vi "Camera.vi"() -> ()   [LabVIEW 2016]
uses:
  <vilib>/rvi/Emulation/niFpgaGetClockAttributes.vi
  <vilib>/rvi/Emulation/niFpgaSctlEmulationGetInTimedLoop.vi
  <vilib>/rvi/Emulation/niFpgaEmulationReportErrorSimple.vi
  <vilib>/rvi/eio/common/nirviEmuTemplateMethod_errors.vi
  <vilib>/rvi/Emulation/niFpgaCriticalErrorInLSC.vi
  <vilib>/eio/EIONode/EIONode.xnode
panel:
  in  "Tlow = t":i16=9
  in  "Fly View Frame Rate = R":i16=10
  in  "Arena View Frame Rate = R":i16=200
  out "Camera flash time":i16
  in  "Camera flash time t":i16
  in  "Flash":bool
  # "** Frequency  = 1 / (Fly View R * 0.0001)   i.e R = 10, Frequency = 1000Hz"
  # "**T period = R*100µs,      T low = t*100 µs"
  # "** Frequency  = 1 / (R * 0.0001)   i.e R = 100, Frequency = 100Hz"
  # "** Trigger the fluorenscence camera (Arena View R - x ) *100 microseconds earlier\n      i.e Arena View R = 100, x = 98,\n           offset x = (100 - 98) * 100 µs = 200 µs"
  # "** Camera flash time is set to be the time for triggering the flash at the end of every video.\n** The unit is second."
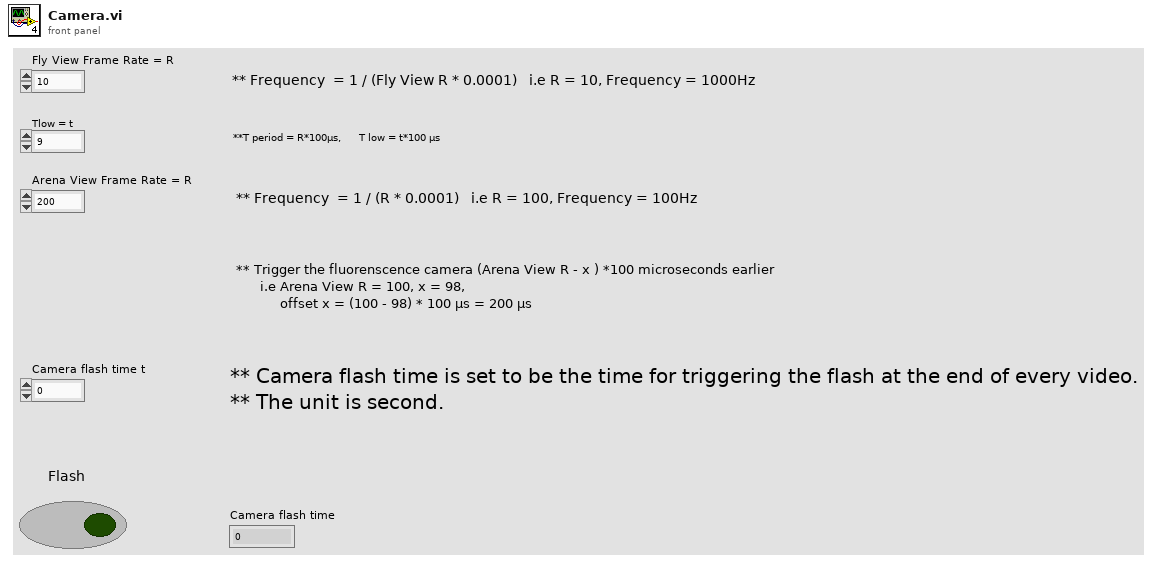
[diagram p1: front panel]
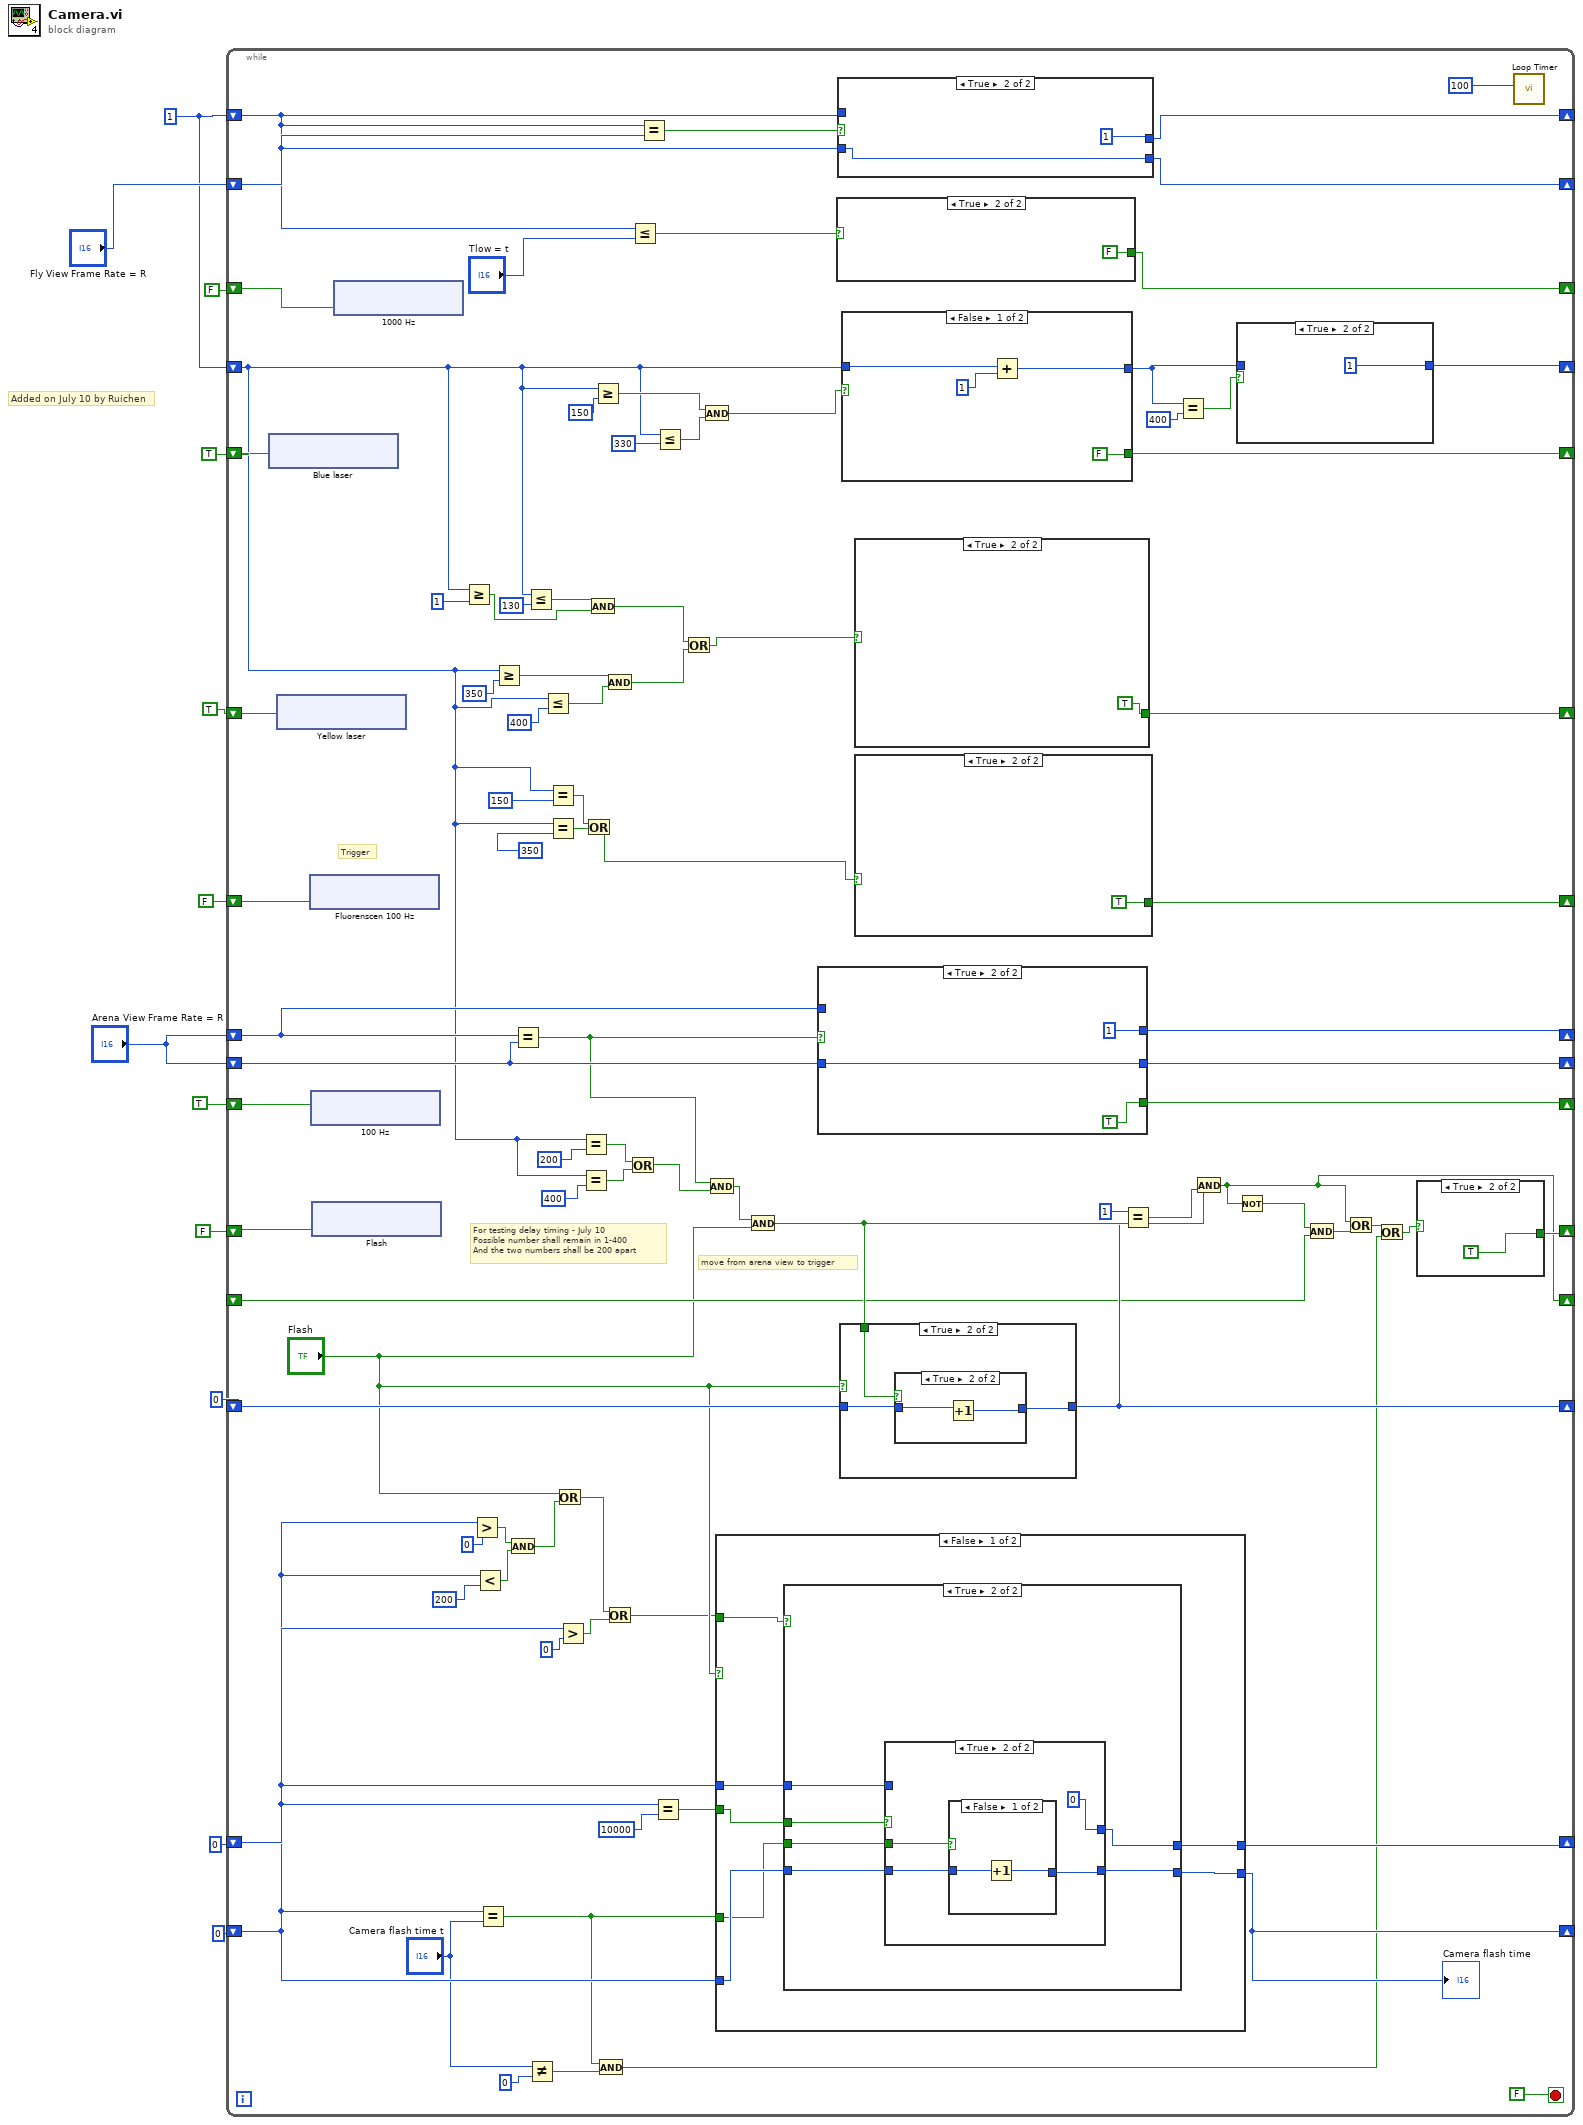
[diagram p0: block diagram]
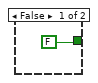
[diagram p2: hidden frame]
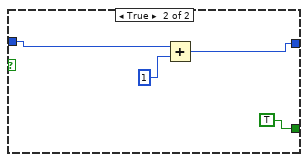
[diagram p4: hidden frame]
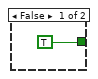
[diagram p5: hidden frame]
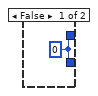
[diagram p6: hidden frame]
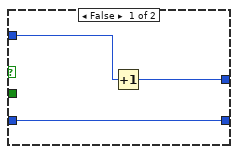
[diagram p7: hidden frame]
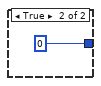
[diagram p8: hidden frame]
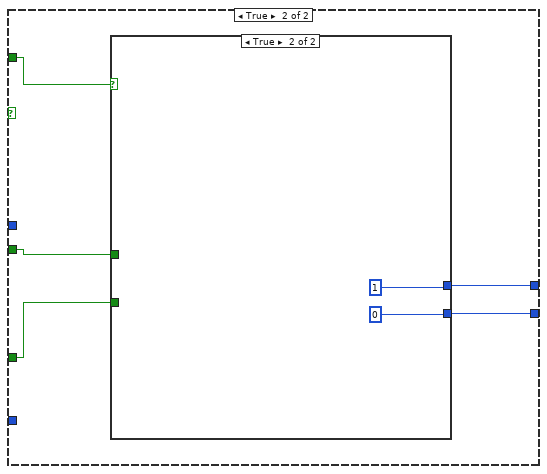
[diagram p9: hidden frame]
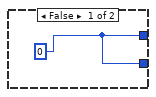
[diagram p10: hidden frame]
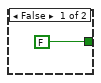
[diagram p11: hidden frame]
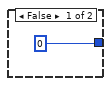
[diagram p12: hidden frame]
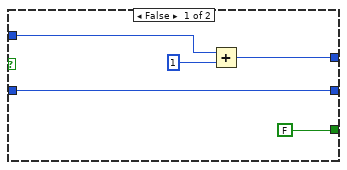
[diagram p14: hidden frame]
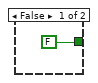
[diagram p15: hidden frame]
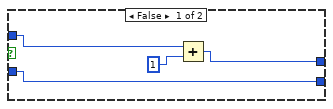
[diagram p16: hidden frame]
diagram:
  w1 = i16 1
  # "Added on July 10 by Ruichen"
  n1 = while {
    shift-right: [w54] -> _
    shift-left: FALSE -> [w102]
    shift-right: [w100] -> _
    shift-left: w1 -> [w50]
    shift-right: [w98] -> _
    shift-left: FALSE -> [w99]
    shift-right: [w97] -> _
    shift-left: TRUE -> [w93]
    shift-right: [w96] -> _
    shift-left: "Arena View Frame Rate = R" -> [w88]
    shift-right: [w90] -> _
    shift-left: i16 0 -> [w94]
    shift-right: [w86] -> _
    shift-left: FALSE -> [w87]
    shift-right: [w82] -> _
    shift-left: _ -> [w83]
    shift-right: [w76] -> _
    shift-left: i16 0 -> [w69]
    shift-right: [w77] -> _
    shift-left: i16 0 -> [w63]
    shift-right: [w57] -> _
    shift-left: "Arena View Frame Rate = R" -> [w56]
    shift-right: [w55] -> _
    shift-left: "Fly View Frame Rate = R" -> [w53]
    shift-right: [w45] -> _
    shift-left: w1 -> [w16]
    shift-right: [w48] -> _
    shift-left: TRUE -> [w49]
    shift-right: [w42] -> _
    shift-left: TRUE -> [w43]
    stop <- FALSE stop-if-true
    # "For testing delay timing - July 10\nPossible number shall remain in 1-400\nAnd the two numbers shall be 200 apart"
    # "move from arena view to trigger"
    # "Trigger"
    n2 = xnode "Blue laser"("ConnectorC/DIO4"=w49) -> ()  [unwired: 1 in, 1 out]
    n3 = xnode "Yellow laser"("ConnectorC/DIO5"=w43) -> ()  [unwired: 1 in, 1 out]
    n4 = xnode "Fluorenscen 100 Hz"("ConnectorC/DIO1"=w99) -> ()  [unwired: 1 in, 1 out]
    n5 = xnode "100 Hz"("ConnectorC/DIO2"=w93) -> ()  [unwired: 1 in, 1 out]
    n6 = xnode "Flash"("ConnectorC/DIO3"=w87) -> ()  [unwired: 1 in, 1 out]
    n7 = xnode "1000 Hz"("ConnectorC/DIO0"=w102) -> ()  [unwired: 1 in, 1 out]
    n8 = Greater Or Equal?(x=w16, y=i16 1) -> (x >= y?=w28:bool)
    n9 = Greater?(x=w63, y=i16 0) -> (0:w66:bool)
    n10 = Less?(x=w63, y=i16 200) -> (x < y?=w65:bool)
    n11 = Equal?(x=w63, y="Camera flash time t") -> (x = y?=w59:bool)
    n12 = Greater Or Equal?(x=w16, y=i16 350) -> (x >= y?=w31:bool)
    n13 = And(x=w66, y=w65) -> (x .and. y?=w64:bool)
    n14 = Equal?(x=w88, y=w56) -> (x = y?=w15:bool)
    n15 = Less Or Equal?(x=w16, y=i16 130) -> (x <= y?=w29:bool)
    n16 = Not Equal?(x="Camera flash time t", y=i16 0) -> (x != y?=w60:bool)
    n17 = Less Or Equal?(x=w16, y=i16 400) -> (x <= y?=w32:bool)
    n18 = Equal?(x=w16, y=i16 150) -> (x = y?=w40:bool)
    n19 = Equal?(x=w16, y=i16 350) -> (x = y?=w38:bool)
    n20 = Or(x="Flash", y=w64) -> (x .or. y?=w71:bool)
    n21 = Greater?(x=w69, y=i16 0) -> (0:w72:bool)
    n22 = Equal?(x=w16, y=i16 200) -> (x = y?=w18:bool)
    n23 = Equal?(x=w16, y=i16 400) -> (x = y?=w17:bool)
    n24 = Or(x=w40, y=w38) -> (x .or. y?=w21:bool)
    n25 = And(x=w29, y=w28) -> (x .and. y?=w27:bool)
    n26 = Greater Or Equal?(x=w16, y=i16 150) -> (x >= y?=w24:bool)
    n27 = And(x=w59, y=w60) -> (x .and. y?=w58:bool)
    n28 = And(x=w31, y=w32) -> (x .and. y?=w30:bool)
    n29 = Or(x=w71, y=w72) -> (x .or. y?=w70:bool)
    n30 = Or(x=w18, y=w17) -> (x .or. y?=w14:bool)
    n31 = Less Or Equal?(x=w50, y="Tlow = t") -> (x <= y?=w52:bool)
    n32 = Equal?(x=w50, y=w53) -> (x = y?=w95:bool)
    n33 = Equal?(x=w69, y=i16 10000) -> (x = y?=w75:bool)
    n34 = Less Or Equal?(x=w16, y=i16 330) -> (x <= y?=w23:bool)
    n35 = Or(x=w27, y=w30) -> (x .or. y?=w37:bool)
    n36 = And(x=w24, y=w23) -> (x .and. y?=w22:bool)
    n37 = And(x=w15, y=w14) -> (x .and. y?=w13:bool)
    n38 = case shown="False" "Flash" {
      tunnel: [w122 w145] -> w77
      tunnel: [w123 w144] -> w76
      tunnel: w69 -> [w120 _]
      tunnel: w75 -> [w121 w143]
      tunnel: w59 -> [w117 w142]
      tunnel: w63 -> [w119 _]
      tunnel: w70 -> [w118 w141]
      frame False {
        n39 = case shown="True" w118 {
          tunnel: [w124 w128] -> w123
          tunnel: [w124 w127] -> w122
          tunnel: w121 -> [_ w130]
          tunnel: w120 -> [_ w129]
          tunnel: w119 -> [_ w126]
          tunnel: w117 -> [_ w125]
          frame False {
            w124 = i16 0
          }
          frame True {
            n40 = case shown="True" w130 {
              tunnel: w129 -> [w133 _]
              tunnel: [w132 i16 0] -> w128
              tunnel: [w131 w136] -> w127
              tunnel: w126 -> [w131 w135]
              tunnel: w125 -> [_ w134]
              frame False {
                n41 = Increment(x=w133) -> (x+1=w132:i16)
              }
              frame True {
                n42 = case shown="False" w134 {
                  tunnel: [w138 i16 0] -> w136
                  tunnel: w135 -> [w139 _]
                  frame False {
                    n43 = Increment(x=w139) -> (x+1=w138:i16)
                  }
                  frame True {
                  }
                }
              }
            }
          }
        }
      }
      frame True {
        n44 = case shown="True" w141 {
          tunnel: [w146 i16 1] -> w144
          tunnel: w142 -> [_ _]
          tunnel: [w146 i16 0] -> w145
          tunnel: w143 -> [_ _]
          frame False {
            w146 = i16 0
          }
          frame True {
          }
        }
      }
    }
    "Camera flash time" <- w77
    n45 = And(x=w13, y="Flash") -> (x .and. y?=w92:bool)
    n46 = case shown="True" w15 {
      tunnel: [FALSE TRUE] -> w97
      tunnel: [w160 i16 1] -> w96
      tunnel: w88 -> [w162 _]
      tunnel: [w158 w163] -> w57
      tunnel: w56 -> [w158 w163]
      frame False {
        n47 = Add(x=w162, y=i16 1) -> (x+y=w160:i16)
      }
      frame True {
      }
    }
    n48 = case shown="True" w52 {
      tunnel: [TRUE FALSE] -> w54
      frame False {
      }
      frame True {
      }
    }
    n49 = case shown="True" w95 {
      tunnel: [w170 i16 1] -> w100
      tunnel: w50 -> [w169 _]
      tunnel: [w168 w172] -> w55
      tunnel: w53 -> [w168 w172]
      frame False {
        n50 = Add(x=w169, y=i16 1) -> (x+y=w170:i16)
      }
      frame True {
      }
    }
    n51 = case shown="True" "Flash" {
      tunnel: w94 -> [_ w153]
      tunnel: [i16 0 w152] -> w90
      tunnel: w92 -> [_ w154]
      frame False {
      }
      frame True {
        n52 = case shown="True" w154 {
          tunnel: w153 -> [w155 w157]
          tunnel: [w155 w156] -> w152
          frame False {
          }
          frame True {
            n53 = Increment(x=w157) -> (x+1=w156:i16)
          }
        }
      }
    }
    n54 = case shown="False" w22 {
      tunnel: w16 -> [w109 w112]
      tunnel: [w108 w111] -> w44
      tunnel: [FALSE TRUE] -> w48
      frame False {
        n55 = Add(x=w109, y=i16 1) -> (x+y=w108:i16)
      }
      frame True {
        n56 = Add(x=w112, y=i16 1) -> (x+y=w111:i16)
      }
    }
    n57 = case shown="True" w37 {
      tunnel: [FALSE TRUE] -> w42
      frame False {
      }
      frame True {
      }
    }
    n58 = case shown="True" w21 {
      tunnel: [FALSE TRUE] -> w98
      frame False {
      }
      frame True {
      }
    }
    n59 = Equal?(x=i16 1, y=w90) -> (x = y?=w89:bool)
    n60 = Equal?(x=w44, y=i16 400) -> (x = y?=w46:bool)
    n61 = And(x=w92, y=w89) -> (x .and. y?=w82:bool)
    n62 = case shown="True" w46 {
      tunnel: [w105 i16 1] -> w45
      tunnel: w44 -> [w105 _]
      frame False {
      }
      frame True {
      }
    }
    n63 = Not(x=w82) -> (.not. x?=w84:bool)
    n64 = And(x=w84, y=w83) -> (x .and. y?=w85:bool)
    n65 = Or(x=w82, y=w85) -> (x .or. y?=w80:bool)
    n66 = Or(x=w80, y=w58) -> (x .or. y?=w79:bool)
    n67 = case shown="True" w79 {
      tunnel: [FALSE TRUE] -> w86
      frame False {
      }
      frame True {
      }
    }
    n68 = call "Loop Timer"("Count(uSec)"=u32 100) -> ()  [unwired: 1 out]
  }
